vi "Create Express VI Terminals.vi"(6 "Terminal Configs":T2[](array[typedef]), 8 "error in (no error)":errorcluster, 11 "Refs in":T1) -> (0 "error out":errorcluster, 3 "Refs":T1)   [LabVIEW 2020, in "FlexBlocks.lvlib"]
uses:
  FlexBlocks.lvlib
  Terminal Config.ctl
  Type Descriptor.ctl
  Terminal Direction.ctl
  Value Mode.ctl
  Special Terminal.ctl
  Terminal Mode.ctl
  Scripting Refs.ctl
  67006990-c909-4462-bc31-5e644962b2dc.vi
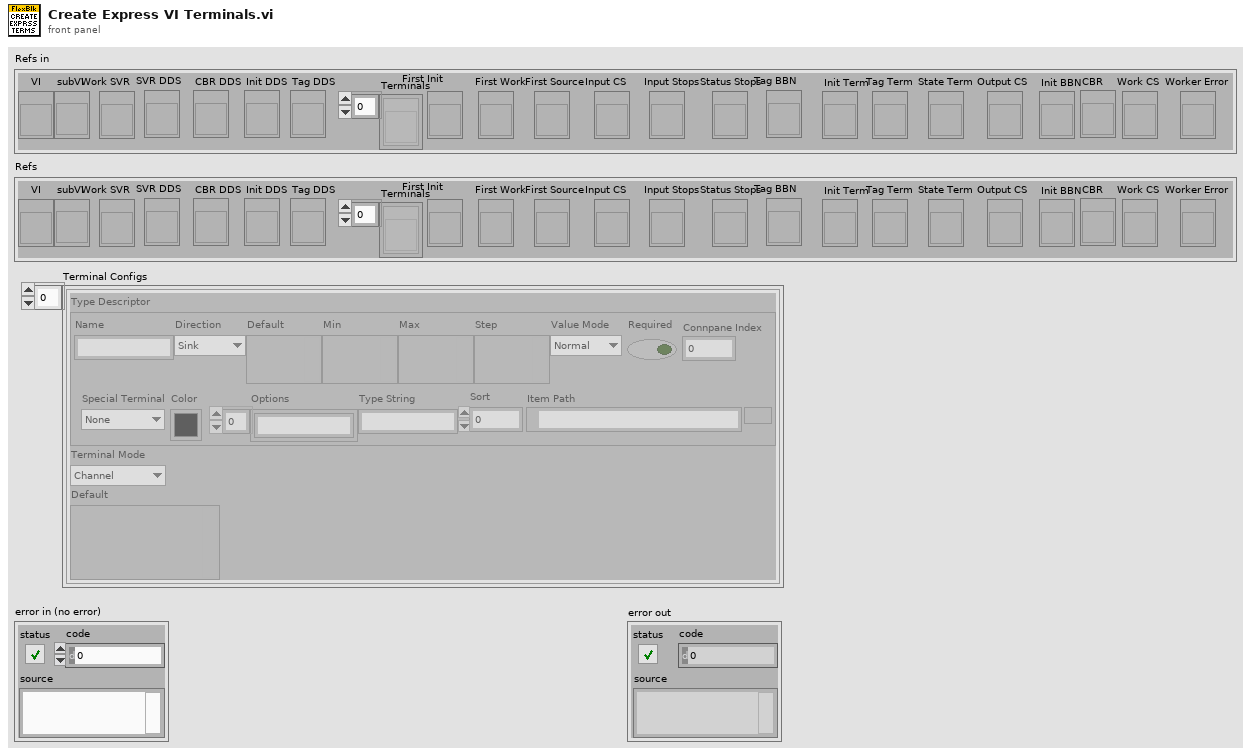
[diagram p1: front panel]
types:
  T1 = typedef "FlexBlocks.lvlib/Scripting Refs.ctl" = cluster{"VI":refnum<vi>, "subVI":refnum<vi>, "Work SVR":refnum<vi>, "SVR DDS":refnum<vi>, "CBR DDS":refnum<vi>, "Init DDS":refnum<vi>, "Tag DDS":refnum<vi>, "Terminals":refnum<vi>[], "First Init":refnum<vi>, "First Work":refnum<vi>, "First Source":refnum<vi>, "Input CS":refnum<vi>, "Input Stops":refnum<vi>, "Status Stops":refnum<vi>, "Tag BBN":refnum<vi>, "Init Term":refnum<vi>, "Tag Term":refnum<vi>, "State Term":refnum<vi>, "Output CS":refnum<vi>, "Init BBN":refnum<vi>, "CBR":refnum<vi>, "Work CS":refnum<vi>, "Worker Error":refnum<vi>}
  T2 = typedef "FlexBlocks.lvlib/Terminal Config.ctl" = cluster{"Type Descriptor":T3, "Terminal Mode":T7, "Default":variant}
  T3 = typedef "FlexBlocks.lvlib/Type Descriptor.ctl" = cluster{"Name":string, "Direction":T4, "Default":variant, "Min":variant, "Max":variant, "Step":variant, "Value Mode":T5, "Required":bool, "Connpane Index":i32, "Special Terminal":T6, "Color":u32, "Options":string[], "Type String":string, "Sort":i32, "Item Path":path}
  T4 = typedef "FlexBlocks.lvlib/Terminal Direction.ctl" = enum16{"Sink", "Source"}
  T5 = typedef "FlexBlocks.lvlib/Value Mode.ctl" = enum16{"Normal", "Range", "Select"}
  T6 = typedef "FlexBlocks.lvlib/Special Terminal.ctl" = enum16{"None", "Action", "Init", "Tag", "State in", "State out", "Error"}
  T7 = typedef "FlexBlocks.lvlib/Terminal Mode.ctl" = enum16{"Channel", "Config", "Value", "Control Ref"}
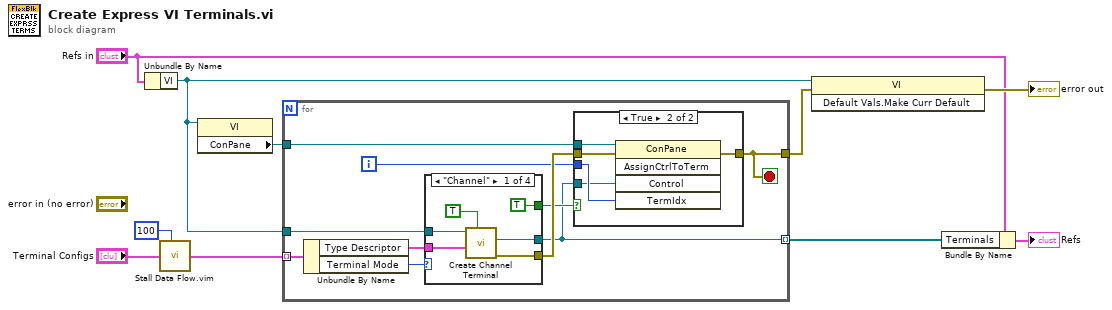
[diagram p0: block diagram]
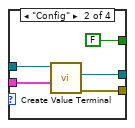
[diagram p2: hidden frame]
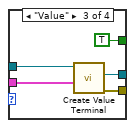
[diagram p3: hidden frame]
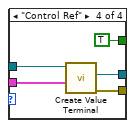
[diagram p4: hidden frame]
diagram:
  n1 = Unbundle By Name("Refs in") -> ("VI"=w6:refnum<vi>)
  n2 = call "Stall Data Flow.vim"("value in"="Terminal Configs", "milliseconds to wait"=u32 100) -> ("value out"=w2:T2[])  [unwired: 1 out]
  n3 = property class="VI"(reference=w6) -> ("ConPane"=w9:refnum<vi>)  [unwired: 1 in, 2 out]
  n4 = for {
    tunnel: w2 -> [w14] mode=indexing
    tunnel: w9 -> [w19]
    tunnel: [w17] -> w7
    tunnel: w6 -> [w15]
    tunnel: [w11] -> w4 mode=indexing
    i -> [w18]
    stop <- w17 stop-if-true
    n5 = Unbundle By Name(w14) -> ("Type Descriptor"=w13:T3, "Terminal Mode"=w16:T7)
    n6 = case shown="\"Channel\"" w16 {
      tunnel: [TRUE FALSE TRUE TRUE] -> w12
      tunnel: w15 -> [w25 w30 w35 w40]
      tunnel: w13 -> [w24 w29 w34 w39]
      tunnel: [w23 w28 w33 w38] -> w11
      tunnel: [w22 w27 w32 w37] -> w20
      frame "Channel" {
        n7 = call "Create Channel Terminal.vi"("Can be Indicator?"=TRUE, "Type Descriptor"=w24, "VI in"=w25) -> ("error out"=w22:errorcluster, "Ctl Refnum"=w23:refnum<vi>)  [unwired: 7 in]
      }
      frame "Config" {
        n8 = call "Create Value Terminal.vi"("Type Descriptor"=w29, "VI in"=w30) -> ("error out"=w27:errorcluster, "Ctl Refnum"=w28:refnum<vi>)  [unwired: 8 in]
      }
      frame "Value" {
        n9 = call "Create Value Terminal.vi"("Type Descriptor"=w34, "VI in"=w35) -> ("error out"=w32:errorcluster, "Ctl Refnum"=w33:refnum<vi>)  [unwired: 8 in]
      }
      frame "Control Ref" {
        n10 = call "Create Value Terminal.vi"("Type Descriptor"=w39, "VI in"=w40) -> ("error out"=w37:errorcluster, "Ctl Refnum"=w38:refnum<vi>)  [unwired: 8 in]
      }
    }
    n11 = case shown="True" w12 {
      tunnel: w19 -> [_ w46]
      tunnel: w18 -> [_ w45]
      tunnel: [_ w44] -> w17
      tunnel: w11 -> [_ w43]
      tunnel: w20 -> [_ w42]
      frame False {
      }
      frame True {
        n12 = invoke class="ConPane" method="AssignCtrlToTerm"(reference=w46, error in=w42, "Control"=w43, "TermIdx"=w45) -> (error out=w44:errorcluster)  [unwired: 1 in, 4 out]
      }
    }
  }
  n13 = invoke class="VI" method="Default Vals.Make Curr Default"(reference=w6, error in=w7) -> (error out=→"error out":errorcluster)  [unwired: 1 in, 2 out]
  n14 = Bundle By Name(cluster="Refs in", "Terminals"=w4) -> (→"Refs":T1)
